vi "Pre Launch Init.vi"(11 "Task Actor in":refnum<class "Task Actor.lvclass">) -> (0 "error out":errorcluster, 3 "Task Actor out":refnum<class "Task Actor.lvclass">)   [LabVIEW 2023, in "Task Actor.lvlib" / "Task Actor.lvclass"]
doc: "(<B>Filename</B>: Actor Framework.lvlib:Actor.lvclass:Pre Launch Init.vi)\n\nDefines behavior that occurs after the Launch Nested Actor method is invoked but before the actor's Actor Core method begins running.\n\nBy default, this method does nothing. A descendant class may override it to define behavior."
uses:
  Task Actor.lvclass
  Task Actor.lvclass/Task Actor.ctl
  Task Base/Task Base.lvclass/Task Base.ctl
  <vilib>/ActorFramework/Actor/Actor.lvclass
  Task Base/Task Base.lvclass
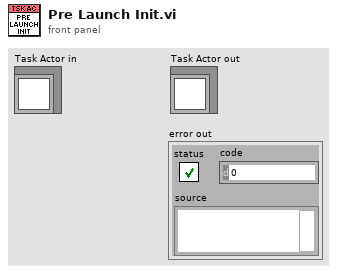
[diagram p1: front panel]
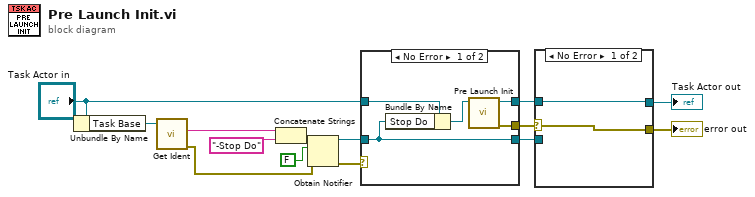
[diagram p0: block diagram]
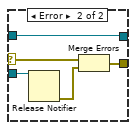
[diagram p2: hidden frame]
diagram:
  n1 = Unbundle By Name("Task Actor in") -> ("Task Base"=w3:refnum<class "Task Base.lvclass">)
  n2 = call "Get Ident.vi"("Task Base in"=w3) -> ("error out"=w1:errorcluster, "Ident"=w2:string)  [unwired: 8 in, 1 out]
  n3 = Concatenate Strings(w2, "-Stop Do" ("name (unnamed)")) -> (w4:string)
  n4 = Obtain Notifier(name (unnamed)=w4, notification data type=FALSE, error in (no error)=w1) -> (notifier out=w7:refnum<notifier>, error out=w12:errorcluster)  [unwired: 1 in, 1 out]
  n5 = case shown="No Error" w12 {
    selector: w12 -> [_ w22]
    tunnel: [w19 w22] -> w11
    tunnel: [w18 w20] -> w10
    tunnel: "Task Actor in" -> [w17 w20]
    tunnel: w7 -> [w15 w21]
    tunnel: [w15 w21] -> w6
    frame No Error {
      n6 = Bundle By Name(cluster=w17, "Stop Do"=w15) -> (w16:refnum<class "Task Actor.lvclass">)
      n7 = call-parent "Pre Launch Init.vi"("Actor in"=w16) -> ("error out"=w19:errorcluster, "Actor out"=w18:refnum<class "Task Actor.lvclass">)  [unwired: 9 in]
    }
    frame Error {
    }
  }
  n8 = case shown="No Error" w11 {
    selector: w11 -> [w23 w27]
    tunnel: w10 -> [w24 w28]
    tunnel: [w24 w28] -> w9
    tunnel: [w23 w29] -> w8
    tunnel: w6 -> [_ w25]
    frame No Error {
    }
    frame Error {
      n9 = Release Notifier(notifier=w25) -> (error out=w26:errorcluster)  [unwired: 2 in, 2 out]
      n10 = Merge Errors(w27, w26) -> (w29:errorcluster)
    }
  }
  "error out" <- w8
  "Task Actor out" <- w9
